vi "config GWS SRM force type.vi"(9 "extension (w/o period)":string="ext1", 10 "typeString (type/subtype)":string="type/subtype", 11 "Configuration String In":string) -> (3 "Modified Configuration":string)   [LabVIEW 2011]
uses:
  <vilib>/regexp/Match Regular Expression.xnode
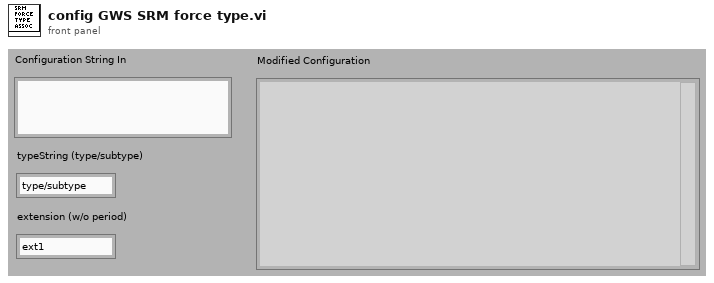
[diagram p1: front panel]
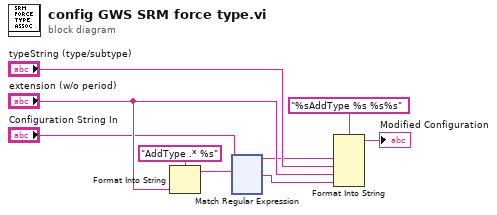
[diagram p0: block diagram]
diagram:
  n1 = Format Into String(format string="AddType .* %s" ("regular expression"), "extension (w/o period)") -> (resulting string=w8:string)  [unwired: 2 in, 1 out]
  n2 = xnode "Match Regular Expression"("input string"="Configuration String In", "regular expression"=w8) -> ("before match"=w4:string, "after match"=w3:string)  [unwired: 4 in, 3 out]
  n3 = Format Into String(format string="%sAddType %s %s%s" ("regular expression"), w4, "typeString (type/subtype)", "extension (w/o period)", w3) -> (resulting string=→"Modified Configuration":string)  [unwired: 2 in, 1 out]
